vi "Connection Callback.vi"(7 "Owner":refnum<class>, 10 "Connection State":T1, 11 "Endpoint":refnum<class "Endpoint.lvclass">) -> ()   [LabVIEW 2020, in "LV Chat Server.lvclass"]
uses:
  LV Chat Server.lvclass
  <vilib>/IlluminatedG/lv-stream/Connection State.ctl
  Stream-Simple-Msg/Endpoint/Endpoint.lvclass
  <vilib>/IlluminatedG/lv-stream/Stream.lvlib
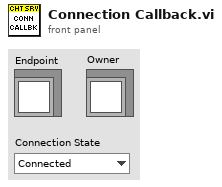
[diagram p1: front panel]
types:
  T1 = typedef "Stream.lvlib/Connection State.ctl" = enum16{"Connected", "Disconnected"}
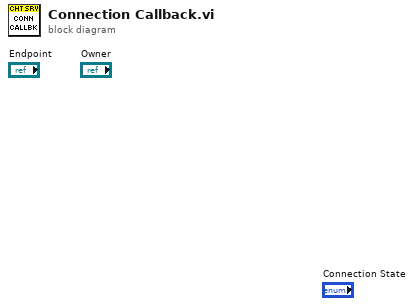
[diagram p0: block diagram]
diagram:
